vi "processNextTask.vi"(8 "error in (no error)":errorcluster, 11 "BuildWorker in":refnum<class "BuildWorker.lvclass">) -> (0 "error out":errorcluster, 3 "BuildWorker out":refnum<class "BuildWorker.lvclass">)   [LabVIEW 2017, in "BuildWorker.lvlib" / "BuildWorker.lvclass"]
uses:
  BuildWorker.lvclass
  C:/Program Files (x86)/National Instruments/LabVIEW 2017/vi.lib/ActorFramework/Actor/Actor.lvclass
  <vilib>/ActorFramework/Actor/Actor.lvclass/Actor.ctl
  <vilib>/ActorFramework/Message Enqueuer/Message Enqueuer.lvclass/Message Enqueuer.ctl
  BuildWorker.lvclass/BuildWorker.ctl
  Classes/Task Interface/Task/Task.lvclass/Task.ctl
  Classes/Task Interface/Task/Status.ctl
  <vilib>/Utility/error.llb/DialogType.ctl
  Classes/Task Interface/Task/Get Name.vi
  <vilib>/ActorFramework/Message Enqueuer/Init from Existing Queue.vi
  <vilib>/ActorFramework/Message Enqueuer/Enqueue.vi
  <vilib>/ActorFramework/Stop Msg/Stop Msg.lvclass
  C:/Program Files (x86)/National Instruments/LabVIEW 2017/vi.lib/ActorFramework/Message/Message.lvclass
  <vilib>/ActorFramework/Message Priority Queue/Priority Enqueue.vi
  <vilib>/ActorFramework/Message Enqueuer/Message Enqueuer.lvclass
  <vilib>/ActorFramework/Actor/Actor.lvclass
  BuildWorker Messages/Send Status Update Msg/Send Status Update Msg.lvclass
  BuildWorker Messages/Update Current Task Name Msg/Update Current Task Name Msg.lvclass
  BuildWorker Messages/Send Task Status Update Msg/Send Task Status Update Msg.lvclass
  BuildWorker Messages/Send Task Outputs Msg/Send Task Outputs Msg.lvclass
  Classes/Task Interface/Task/Task.lvclass
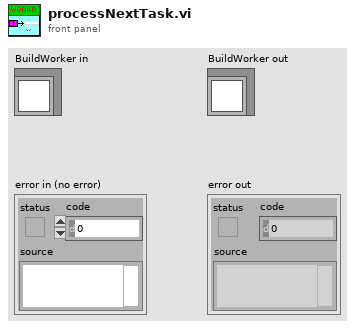
[diagram p1: front panel]
types:
  T1 = typedef "Task Interface.lvlib/Task.lvclass/Status.ctl" = enum16{"Created", "Added", "Pending", "Queued", "Processing", "Cleaning", "Building", "Finished", "Failed", "Removed", "Not found"}
  T2 = typedef "NI_App_Builder_API.lvlib/Build Specification Version.ctl" = cluster{"Major":u16, "Minor":u16, "Fix":u16, "Build":u16}
  T3 = typedef "DialogType.ctl" = u16
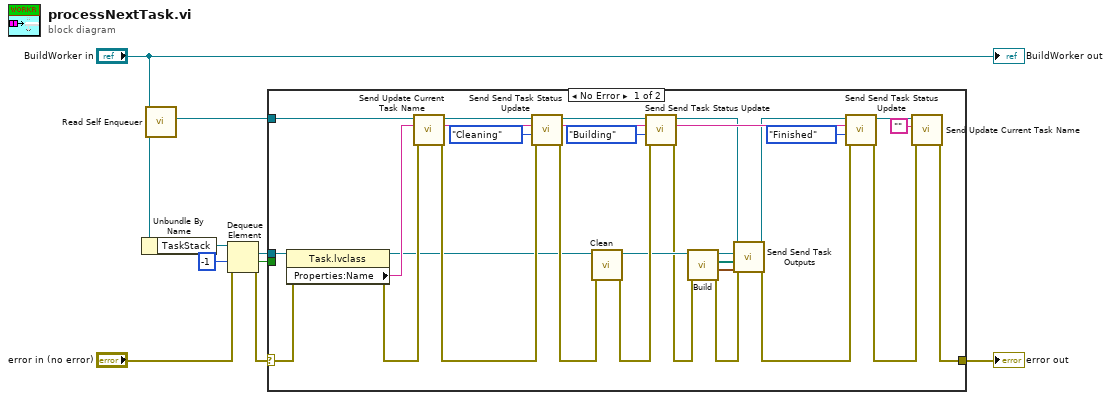
[diagram p0: block diagram]
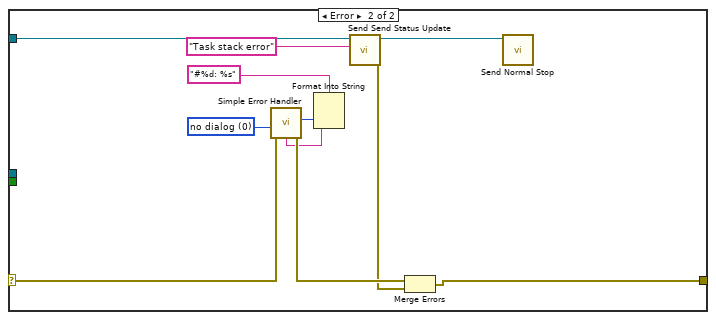
[diagram p2: hidden frame]
diagram:
  n1 = Unbundle By Name("BuildWorker in") -> ("TaskStack"=w6:refnum<queue>)
  n2 = call <vilib>:"Read Self Enqueuer.vi"("Actor"="BuildWorker in") -> ("Self Enqueuer"=w5:refnum<class "Message Enqueuer.lvclass">)  [unwired: 10 in]
  n3 = Dequeue Element(queue=w6, timeout in ms (-1)=-1, error in (no error)="error in (no error)") -> (element=w7:refnum<class "Task.lvclass">, timed out?=w1:bool, error out=w3:errorcluster)  [unwired: 1 out]
  n4 = case shown="No Error" w3 {
    selector: w3 -> [w32 w45]
    tunnel: w7 -> [w36 _]
    tunnel: w5 -> [w31 w47]
    tunnel: [w23 w39] -> w4
    tunnel: w1 -> [_ _]
    frame No Error {
      n5 = property class="Task.lvclass"(reference=w36, error in=w32) -> (reference out=w26:refnum<class "Task.lvclass">, error out=w27:errorcluster, "Properties:Name"=w28:string)
      n6 = call "Send Update Current Task Name.vi"("error in (no error)"=w27, "CurrentTaskName"=w28, "Message Enqueuer in"=w31) -> ("error out"=w29:errorcluster, "Message Enqueuer out"=w30:refnum<class "Message Enqueuer.lvclass">)  [unwired: 7 in]
      n7 = call "Send Send Task Status Update.vi"("error in (no error)"=w29, "Status"=Status."Cleaning", "Task Name"=w28, "Message Enqueuer in"=w30) -> ("error out"=w35:errorcluster, "Message Enqueuer out"=w34:refnum<class "Message Enqueuer.lvclass">)  [unwired: 6 in]
      n8 = call "Clean.vi"("error in (no error)"=w35, "Task in"=w26) -> ("error out"=w33:errorcluster, "Task out"=w18:refnum<class "Task.lvclass">)  [unwired: 8 in]
      n9 = call "Send Send Task Status Update.vi"("error in (no error)"=w33, "Status"=Status."Building", "Task Name"=w28, "Message Enqueuer in"=w34) -> ("error out"=w17:errorcluster, "Message Enqueuer out"=w11:refnum<class "Message Enqueuer.lvclass">)  [unwired: 6 in]
      n10 = call "Build.vi"("error in (no error)"=w17, "Task in"=w18) -> ("error out"=w13:errorcluster, "Build Specification Version"=w14:T2, "Generated files"=w15:path[], "Task out"=w16:refnum<class "Task.lvclass">)  [unwired: 6 in]
      n11 = call "Send Send Task Outputs.vi"("Build Specification Version"=w14, "error in (no error)"=w13, "Generated files"=w15, "Task"=w16, "Message Enqueuer in"=w11) -> ("error out"=w12:errorcluster, "Message Enqueuer out"=w10:refnum<class "Message Enqueuer.lvclass">)  [unwired: 5 in]
      n12 = call "Send Send Task Status Update.vi"("error in (no error)"=w12, "Status"=Status."Finished", "Task Name"=w28, "Message Enqueuer in"=w10) -> ("error out"=w24:errorcluster, "Message Enqueuer out"=w25:refnum<class "Message Enqueuer.lvclass">)  [unwired: 6 in]
      n13 = call "Send Update Current Task Name.vi"("error in (no error)"=w24, "CurrentTaskName"="", "Message Enqueuer in"=w25) -> ("error out"=w23:errorcluster)  [unwired: 7 in, 1 out]
    }
    frame Error {
      w43 = T3 0 items=["no dialog", "OK message", "continue or stop message", "OK message + warnings", "continue/stop + warnings"] ("type of dialog (OK msg:1)")
      n14 = call <vilib>:"Simple Error Handler.vi"("type of dialog (OK msg:1)"=w43, "error in (no error)"=w45) -> ("code out"=w42:i32, "error out"=w44:errorcluster, "message"=w41:string)  [unwired: 3 in, 2 out]
      n15 = Format Into String(format string="#%d: %s", w42, w41) -> ()  [unwired: 2 in, 2 out]
      n16 = call "Send Send Status Update.vi"("Task Name"="Task stack error", "Message Enqueuer in"=w47) -> ("error out"=w38:errorcluster, "Message Enqueuer out"=w37:refnum<class "Message Enqueuer.lvclass">)  [unwired: 8 in]
      n17 = Merge Errors(w44, w38) -> (w39:errorcluster)
      n18 = call <vilib>:"Send Normal Stop.vi"("Message Enqueuer"=w37) -> ()  [unwired: 10 in, 1 out]
    }
  }
  "error out" <- w4
  "BuildWorker out" <- "BuildWorker in"
